vi "Calculate.vi"(8 "error in (no error)":errorcluster, 9 "Reference Rectangle":T1, 10 "My VI":string, 11 "Static in":refnum<class "Reference Size.lvclass">) -> (0 "error out":errorcluster, 1 "Height":i16, 2 "Width":i16)   [LabVIEW 2020, in "Panel.lvlib" / "Reference Size.lvclass"]
doc: "Calculates the window size\n\n----\nPlease see the following web address for additional documentation and tutorial information:\nhttp://www.mooregoodideas.com/mgi-panel-manager/\n\nAuthor: Derek Trepanier\n\nCopyright (c) 2018, Moore Good Ideas, Inc.\n\nAll rights reserved.\n\nRedistribution and use in source and binary forms, with or without modification, are permitted provided that the following conditions are met:\n\n * Redistributions of source code must retain the above copyright notice, this list of conditions and the following disclaimer.\n * Redistributions in binary form must reproduce the above copyright notice, this list of conditions and the following disclaimer in the documentation and/or other materials provided with the distribution.\n * Neither the name of Moore Good Ideas, Inc. nor the names of its contributors may be used to endorse or promote products derived from this software without specific prior written permission.\n\nTHIS SOFTWARE IS PROVIDED BY THE COPYRIGHT HOLDERS AND CONTRIBUTORS \"AS IS\" AND ANY EXPRESS OR IMPLIED WARRANTIES, INCLUDING, BUT NOT LIMITED TO, THE IMPLIED WARRANTIES OF MERCHANTABILITY AND FITNESS FOR A PARTICULAR PURPOSE ARE DISCLAIMED. IN NO EVENT SHALL THE COPYRIGHT OWNER OR CONTRIBUTORS BE LIABLE FOR ANY DIRECT, INDIRECT, INCIDENTAL, SPECIAL, EXEMPLARY, OR CONSEQUENTIAL DAMAGES (INCLUDING, BUT NOT LIMITED TO, PROCUREMENT OF SUBSTITUTE GOODS OR SERVICES; LOSS OF USE, DATA, OR PROFITS; OR BUSINESS INTERRUPTION) HOWEVER CAUSED AND ON ANY THEORY OF LIABILITY, WHETHER IN CONTRACT, STRICT LIABILITY, OR TORT (INCLUDING NEGLIGENCE OR OTHERWISE) ARISING IN ANY WAY OUT OF THE USE OF THIS SOFTWARE, EVEN IF ADVISED OF THE POSSIBILITY OF SUCH DAMAGE."
uses:
  <vilib>/MGI/Panel Manager/Panel/Window Position/Reference Position/Size/Reference Size/Reference Size.lvclass
  <vilib>/Utility/miscctls.llb/LVRectTypeDef.ctl
  <vilib>/MGI/Panel Manager/Panel/Window Position/Reference Position/Size/Reference Size/Reference Size.lvclass/Reference Size.ctl
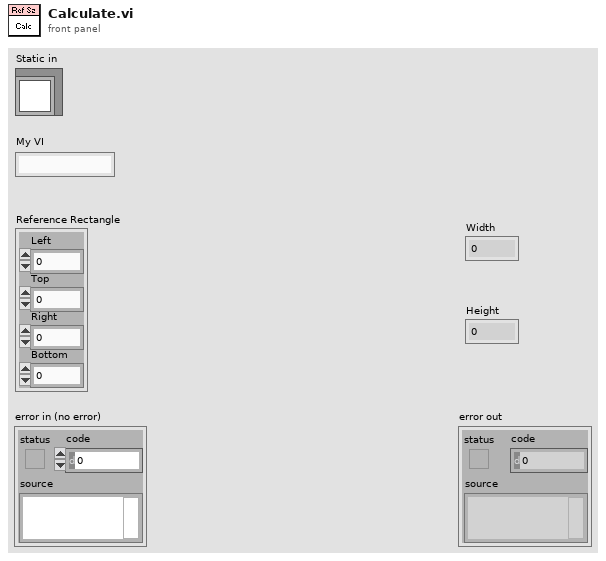
[diagram p1: front panel]
types:
  T1 = typedef "LVRectTypeDef.ctl" = cluster{"Left":i16, "Top":i16, "Right":i16, "Bottom":i16}
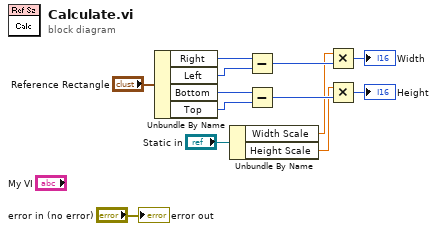
[diagram p0: block diagram]
diagram:
  n1 = Unbundle By Name("Reference Rectangle") -> ("Right"=w12:i16, "Left"=w11:i16, "Bottom"=w10:i16, "Top"=w9:i16)
  n2 = Unbundle By Name("Static in") -> ("Width Scale"=w4:dbl, "Height Scale"=w1:dbl)
  n3 = Subtract(x=w12, y=w11) -> (x-y=w7:i16)
  n4 = Subtract(x=w10, y=w9) -> (x-y=w6:i16)
  n5 = Multiply(x=w4, y=w7) -> (x*y=→"Width":i16)
  n6 = Multiply(x=w1, y=w6) -> (x*y=→"Height":i16)
  "error out" <- "error in (no error)"
